vi "GetText.vi"(8 "error in":errorcluster, 11 "Tag Bus Web Interface editor node in":refnum<class "Tag Bus Web Interface editor node.lvclass">) -> (0 "error out":errorcluster, 1 "additional text":string, 2 "text":string, 3 "Tag Bus Web Interface editor node out":refnum<class "Tag Bus Web Interface editor node.lvclass">, 4 "glyph":string)   [LabVIEW 2013, in "Tag Bus Web Interface editor node.lvclass"]
uses:
  Tag Bus Web Interface editor node.lvclass
  <vilib>/NI/Tag Bus Data Framework/Configuration Editor/Classes/Module editor node/module editor node.lvclass
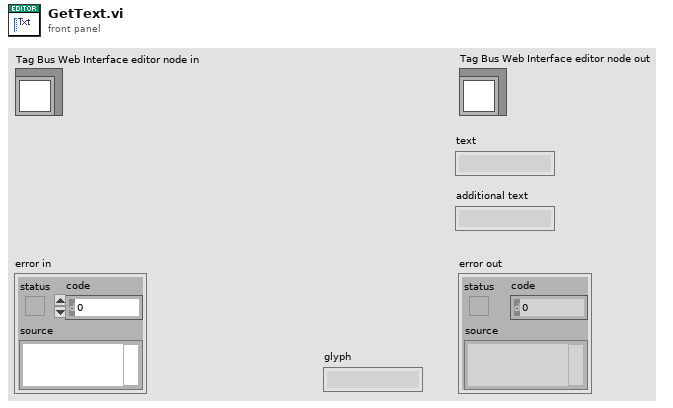
[diagram p1: front panel]
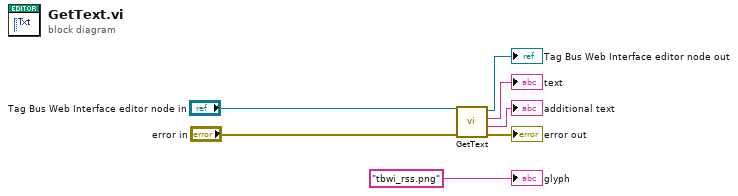
[diagram p0: block diagram]
diagram:
  n1 = call-parent "GetText.vi"("error in"="error in", "Module Editor Node in"="Tag Bus Web Interface editor node in") -> ("error out"=→"error out":errorcluster, "additional text"=→"additional text":string, "text"=→"text":string, "Module Editor Node out"=→"Tag Bus Web Interface editor node out":refnum<class "Tag Bus Web Interface editor node.lvclass">)  [unwired: 5 in, 1 out]
  "glyph" <- "tbwi_rss.png" ("glyph")
